vi "UHR-Fleezers Control (host) - 11.9.vi"() -> ()   [LabVIEW 2014] (continued)
                    tunnel: [w550 w565] -> w545
                    tunnel: w544 -> [_ w561]
                    frame False {
                      n310 = local read "Fish"() -> (w550:bool)
                      n311 = case shown="False" w550 {
                        tunnel: w551 -> [w552 _]
                        frame False {
                          n312 = property on="BD 1 Frequency 1 (MHz)" class="DigNum (strict)"("Val(Sgnl)"=w552) -> ()  [unwired: 2 in, 2 out]
                        }
                        frame True {
                        }
                      }
                    }
                    frame True {
                      w565 = FALSE ("Fish for Tether")
                      n313 = call <vilib>:"Beep.vi"() -> ()  [unwired: 3 in, 9 out]
                      n314 = Number To Decimal String(number=w561, width (-)=i16 1) -> (decimal integer string=w559:string)
                      n315 = Concatenate Strings("Formed tether in ", w559, " attempt(s)." ("string")) -> (w556:string)
                      n316 = local read "Messages"() -> (w563:string)
                      n317 = local write "Fish"(w565) -> ()
                      n318 = call "Update messages.vi"("Message to add"=w556, "Old message string"=w563) -> ("New message string"=w562:string)
                      n319 = local write "Messages"(w562) -> ()
                      n320 = Get Date/Time In Seconds() -> (seconds since 1Jan1904=→"Time tether formed":timestamp)
                      n321 = local read "Flow ON\nduring cal?"() -> (w553:bool)
                      n322 = property on="Sample Channel\nFlow" class="Bool (strict)"("Val(Sgnl)"=w553) -> (error out=w554:errorcluster)  [unwired: 2 in, 1 out]
                      n323 = case shown="\"2\", \"3\", \"4\", \"5\", \"6\"" "Then..." {
                        selector: "Then..." -> [_ w569 _ _]
                        tunnel: w566 -> [w568 _ _ _]
                        tunnel: w554 -> [_ _ _ _]
                        frame "1", Default {
                          n324 = property on="BD 1 Frequency 1 (MHz)" class="DigNum (strict)"("Val(Sgnl)"=w568) -> ()  [unwired: 2 in, 2 out]
                        }
                        frame "2", "3", "4", "5", "6" {
                          n325 = flat-sequence {
                            tunnel: w569 -> [w575]
                            frame #0 {
                              n326 = local read "Flow ON\nduring cal?"() -> (w570:bool)
                              n327 = property on="Sample Channel\nFlow" class="Bool (strict)"("Val(Sgnl)"=w570) -> ()  [unwired: 2 in, 2 out]
                              n328 = property on="Trap D (MHz)" class="DigNum (strict)"("Val(Sgnl)"="Move to D 1 (MHz)") -> ()  [unwired: 2 in, 2 out]
                            }
                            frame #1 {
                              n329 = local read "Wait Before Save (s)"() -> (w572:u32)
                              n330 = Multiply(x=u32 1000 ("milliseconds to wait"), y=w572) -> (x*y=w574:u32)
                              n331 = Wait (ms)(milliseconds to wait=w574) -> ()  [unwired: 1 out]
                            }
                            frame #2 {
                              n332 = case shown="\"5\", \"6\"" w575 {
                                selector: w575 -> [w578 w588 _]
                                frame "3", "4" {
                                n333 = flat-sequence {
                                tunnel: w578 -> [w579]
                                tunnel: [w579] -> w576
                                tunnel: [w581] -> w577
                                tunnel: w576 -> [w581]
                                tunnel: w577 -> [w585]
                                frame #0 {
                                n334 = property on="Green ON/Interlacing" class="Bool (strict)"("Val(Sgnl)"=TRUE ("Value (Signaling)")) -> ()  [unwired: 2 in, 2 out]
                                }
                                frame #1 {
                                n335 = Multiply(x="Wait Before Save (s)", y=u32 1000 ("x")) -> (x*y=w583:u32)
                                n336 = Wait (ms)(milliseconds to wait=w583) -> ()  [unwired: 1 out]
                                }
                                frame #2 {
                                n337 = property on="Start Saving" class="Bool (strict)"("Value"=TRUE ("Start Saving")) -> ()  [unwired: 2 in, 2 out]
                                n338 = case shown="\"4\"" w585 {
                                frame Default {
                                }
                                frame "4" {
                                n339 = property on="Fl. Triggered..." class="Bool (strict)"("Val(Sgnl)"=TRUE ("Value (Signaling)")) -> ()  [unwired: 2 in, 2 out]
                                }
                                }
                                }
                                }
                                }
                                frame "5", "6" {
                                n340 = stacked-sequence {
                                tunnel: w588 -> [_ _ _ _ _ _ w600]
                                frame #0 {
                                n341 = Replace Array Subset(array=u32[] [0] ("Index Values"), new element="Raster Set\nUpon Tether", index=0) -> (w589:u32[])
                                n342 = property on="Saved AOD Raster Scan Parameter Sets" class="Arr (strict)"("Index Values"=w589) -> ()  [unwired: 2 in, 2 out]
                                }
                                frame #1 {
                                n343 = Wait (ms)(milliseconds to wait=u32 500) -> ()  [unwired: 1 out]
                                }
                                frame #2 {
                                n344 = property on="Load parameters" class="Bool (strict)"("Val(Sgnl)"=TRUE ("Value (Signaling)")) -> ()  [unwired: 2 in, 2 out]
                                n345 = case shown="True" "Green ON during\nraster?" {
                                frame False {
                                }
                                frame True {
                                n346 = property on="Green ON/Interlacing" class="Bool (strict)"("Val(Sgnl)"=TRUE ("Value (Signaling)")) -> ()  [unwired: 2 in, 2 out]
                                }
                                }
                                }
                                frame #3 {
                                n347 = Wait (ms)(milliseconds to wait=u32 500) -> ()  [unwired: 1 out]
                                }
                                frame #4 {
                                n348 = property on="Trap Raster Scan" class="Bool (strict)"("Val(Sgnl)"=TRUE ("Value (Signaling)")) -> ()  [unwired: 2 in, 2 out]
                                }
                                frame #5 {
                                n349 = Wait (ms)(milliseconds to wait=u32 2000) -> ()  [unwired: 1 out]
                                }
                                frame #6 {
                                n350 = flat-sequence {
                                tunnel: w600 -> [w607]
                                frame #0 {
                                n351 = while {
                                stop <- w603 stop-if-true
                                n352 = local read "Raster Scanning..."() -> (w602:bool)
                                n353 = local read "Saving..."() -> (w605:bool)
                                n354 = Wait (ms)(milliseconds to wait=u32 100) -> ()  [unwired: 1 out]
                                n355 = Not(x=w605) -> (.not. x?=w604:bool)
                                n356 = Not(x=w602) -> (.not. x?=w601:bool)
                                n357 = And(x=w604, y=w601) -> (x .and. y?=w603:bool)
                                }
                                }
                                frame #1 {
                                n358 = local read "Tether"() -> (w608:bool)
                                n359 = case shown="True" w608 {
                                tunnel: w607 -> [_ w610]
                                frame False {
                                n360 = property on="Fish" class="Bool (strict)"("Val(Sgnl)"="Fish again after \nraster break?") -> ()  [unwired: 2 in, 2 out]
                                }
                                frame True {
                                n361 = stacked-sequence {
                                tunnel: w610 -> [_ w614 _ _ _ _ _ _]
                                frame #0 {
                                n362 = property on="Trap D (MHz)" class="DigNum (strict)"("Val(Sgnl)"="Move to D 2 (MHz)") -> ()  [unwired: 2 in, 2 out]
                                n363 = case shown="True" "Flow ON after\ntether testing?" {
                                frame False {
                                }
                                frame True {
                                n364 = property on="Sample Channel\nFlow" class="Bool (strict)"("Val(Sgnl)"=TRUE ("Value (Signaling)")) -> ()  [unwired: 2 in, 2 out]
                                }
                                }
                                }
                                frame #1 {
                                n365 = flat-sequence {
                                tunnel: w614 -> [w615]
                                frame #0 {
                                n366 = case shown="\"6\"" w615 {
                                frame Default {
                                }
                                frame "6" {
                                n367 = flat-sequence {
                                frame #0 {
                                n368 = Wait (ms)(milliseconds to wait=u32 500) -> ()  [unwired: 1 out]
                                }
                                frame #1 {
                                n369 = property on="Green ON/Interlacing" class="Bool (strict)"("Val(Sgnl)"=TRUE ("Green Laser ON/Interlacing")) -> ()  [unwired: 2 in, 2 out]
                                }
                                }
                                }
                                }
                                }
                                frame #1 {
                                n370 = case shown="True" "Save at end (5, 6)" {
                                selector: "Save at end (5, 6)" -> [_ w619]
                                frame False {
                                }
                                frame True {
                                n371 = flat-sequence {
                                tunnel: w619 -> [w621]
                                frame #0 {
                                n372 = Wait (ms)(milliseconds to wait=u32 500) -> ()  [unwired: 1 out]
                                }
                                frame #1 {
                                n373 = local write "Start Saving"(w621) -> ()
                                }
                                }
                                }
                                }
                                }
                                }
                                }
                                frame #2 {
                                n374 = local read "Bead Sep. Int. Time (s)"() -> (w624:dbl)
                                n375 = Multiply(x=w624, y=1000.0) -> (x*y=w623:dbl)
                                n376 = Wait (ms)(milliseconds to wait=w623) -> ()  [unwired: 1 out]
                                }
                                frame #3 {
                                n377 = property on="Remove Offset" class="Bool (strict)"("Val(Sgnl)"=TRUE ("Value (Signaling)")) -> ()  [unwired: 2 in, 2 out]
                                }
                                frame #4 {
                                n378 = property on="Read FX file" class="Bool (strict)"("Val(Sgnl)"=TRUE ("Value (Signaling)")) -> ()  [unwired: 2 in, 2 out]
                                }
                                frame #5 {
                                n379 = Wait (ms)(milliseconds to wait=u32 300) -> ()  [unwired: 1 out]
                                }
                                frame #6 {
                                n380 = local read "Bad fit error"() -> (w633:dbl)
                                n381 = local read "Fit offset"() -> (w636:dbl)
                                n382 = Greater Or Equal?(x=w633, y="Bad fit thresh") -> (x >= y?=→"Bad fit":bool)
                                n383 = Greater Or Equal?(x=w636, y="Fit offset thresh") -> (x >= y?=→"Multiple tether":bool)
                                n384 = local read "Hyst. error"() -> (w630:dbl)
                                n385 = Greater Or Equal?(x=w630, y="Hysteresis thresh") -> (x >= y?=→"Hysteresis":bool)
                                }
                                frame #7 {
                                w641 = 0
                                n386 = local read "Bad fit error"() -> (w643:dbl)
                                n387 = local read "Hyst. error"() -> (w642:dbl)
                                n388 = local read "Fit offset"() -> (w644:dbl)
                                n389 = local read "Multiple tether"() -> (w650:bool)
                                n390 = local read "Hysteresis"() -> (w648:bool)
                                n391 = local read "Bad fit"() -> (w649:bool)
                                n392 = Not(x=w648) -> (.not. x?=w640:bool)
                                n393 = Not(x=w649) -> (.not. x?=w646:bool)
                                n394 = Greater?(x=w644, y=w641) -> (0:w639:bool)
                                n395 = Greater?(x=w643, y=w641) -> (0:w638:bool)
                                n396 = Greater?(x=w642, y=w641) -> (0:w637:bool)
                                n397 = Not(x=w650) -> (.not. x?=w647:bool)
                                n398 = Compound Arithmetic op=AND(w647, w646, w640, w639, w638, w637) -> (w645:bool)
                                "Good tether" <- w645
                                n399 = case shown="True" w645 {
                                frame False {
                                }
                                frame True {
                                n400 = call <vilib>:"Beep.vi"("use system alert? (T)"=FALSE, "duration (msec)"=u32 200, "frequency (Hz)"=u32 2000) -> ()  [unwired: 9 in]
                                }
                                }
                                }
                                }
                                }
                                }
                                }
                                }
                                }
                                }
                                }
                                frame "2", Default {
                                }
                              }
                            }
                            frame #3 {
                              n401 = local read "Multiple tether"() -> (w656:bool)
                              n402 = And(x="Break multiple", y=w656) -> (x .and. y?=w654:bool)
                              n403 = case shown="True" w654 {
                                frame False {
                                }
                                frame True {
                                n404 = stacked-sequence {
                                frame #0 {
                                n405 = property on="Trap D (MHz)" class="DigNum (strict)"("Val(Sgnl)"="Trap D to \nbreak (MHz)") -> ()  [unwired: 2 in, 2 out]
                                }
                                frame #1 {
                                n406 = case shown="True" "Fish after\nmultiple break" {
                                frame False {
                                }
                                frame True {
                                n407 = while {
                                stop <- w661 stop-if-true
                                n408 = local read "Multiple tether"() -> (w663:bool)
                                n409 = local read "Fish"() -> (w660:bool)
                                n410 = local read "Stop All"() -> (w659:bool)
                                n411 = Wait (ms)(milliseconds to wait=u32 100) -> ()  [unwired: 1 out]
                                n412 = Not(x=w663) -> (.not. x?=w662:bool)
                                n413 = Compound Arithmetic op=OR(w659, w662, w660) -> (w661:bool)
                                }
                                }
                                }
                                }
                                frame #2 {
                                n414 = local read "Fish after\nmultiple break"() -> (w668:bool)
                                n415 = local read "Stage Moving"() -> (w667:bool)
                                n416 = Not(x=w667) -> (.not. x?=w665:bool)
                                n417 = And(x=w668, y=w665) -> (x .and. y?=w666:bool)
                                n418 = property on="Fish" class="Bool (strict)"("Val(Sgnl)"=w666) -> ()  [unwired: 2 in, 2 out]
                                }
                                }
                                }
                              }
                            }
                            frame #4 {
                              n419 = local read "Bad fit"() -> (w670:bool)
                              n420 = And(x="Break bad fit", y=w670) -> (x .and. y?=w669:bool)
                              n421 = case shown="True" w669 {
                                frame False {
                                }
                                frame True {
                                n422 = stacked-sequence {
                                frame #0 {
                                n423 = local read "Trap D to \nbreak (MHz)"() -> (w672:dbl)
                                n424 = property on="Trap D (MHz)" class="DigNum (strict)"("Val(Sgnl)"=w672) -> ()  [unwired: 2 in, 2 out]
                                }
                                frame #1 {
                                n425 = case shown="True" "Fish after\nbad fit break?" {
                                frame False {
                                }
                                frame True {
                                n426 = while {
                                stop <- w676 stop-if-true
                                n427 = local read "Stop All"() -> (w674:bool)
                                n428 = local read "Bad fit"() -> (w675:bool)
                                n429 = local read "Fish"() -> (w677:bool)
                                n430 = Not(x=w675) -> (.not. x?=w678:bool)
                                n431 = Wait (ms)(milliseconds to wait=u32 100) -> ()  [unwired: 1 out]
                                n432 = Compound Arithmetic op=OR(w674, w678, w677) -> (w676:bool)
                                }
                                }
                                }
                                }
                                frame #2 {
                                n433 = local read "Fish after\nbad fit break?"() -> (w680:bool)
                                n434 = local read "Stage Moving"() -> (w683:bool)
                                n435 = Not(x=w683) -> (.not. x?=w682:bool)
                                n436 = And(x=w680, y=w682) -> (x .and. y?=w681:bool)
                                n437 = property on="Fish" class="Bool (strict)"("Val(Sgnl)"=w681) -> ()  [unwired: 2 in, 2 out]
                                }
                                }
                                }
                              }
                            }
                            frame #5 {
                              n438 = local read "Hysteresis"() -> (w685:bool)
                              n439 = And(x="Break hyst", y=w685) -> (x .and. y?=w684:bool)
                              n440 = case shown="True" w684 {
                                frame False {
                                }
                                frame True {
                                n441 = stacked-sequence {
                                frame #0 {
                                n442 = local read "Trap D to \nbreak (MHz)"() -> (w687:dbl)
                                n443 = property on="Trap D (MHz)" class="DigNum (strict)"("Val(Sgnl)"=w687) -> ()  [unwired: 2 in, 2 out]
                                }
                                frame #1 {
                                n444 = case shown="True" "Fish ater hyst?" {
                                frame False {
                                }
                                frame True {
                                n445 = while {
                                stop <- w693 stop-if-true
                                n446 = local read "Hysteresis"() -> (w692:bool)
                                n447 = local read "Stop All"() -> (w689:bool)
                                n448 = local read "Fish"() -> (w690:bool)
                                n449 = Wait (ms)(milliseconds to wait=u32 100) -> ()  [unwired: 1 out]
                                n450 = Not(x=w692) -> (.not. x?=w691:bool)
                                n451 = Compound Arithmetic op=OR(w689, w691, w690) -> (w693:bool)
                                }
                                }
                                }
                                }
                                frame #2 {
                                n452 = local read "Fish ater hyst?"() -> (w698:bool)
                                n453 = local read "Stage Moving"() -> (w697:bool)
                                n454 = Not(x=w697) -> (.not. x?=w696:bool)
                                n455 = And(x=w698, y=w696) -> (x .and. y?=w695:bool)
                                n456 = property on="Fish" class="Bool (strict)"("Val(Sgnl)"=w695) -> ()  [unwired: 2 in, 2 out]
                                }
                                }
                                }
                              }
                            }
                            frame #6 {
                              n457 = local read "Good tether"() -> (w699:bool)
                              n458 = case shown="True" w699 {
                                frame False {
                                }
                                frame True {
                                n459 = case shown="\"1\"" "If good, then:" {
                                frame "0", Default {
                                }
                                frame "1" {
                                n460 = property on="Force FB Script" class="Bool (strict)"("Val(Sgnl)"=TRUE ("Value (Signaling)")) -> ()  [unwired: 2 in, 2 out]
                                }
                                }
                                }
                              }
                            }
                          }
                        }
                        frame "7" {
                          n461 = property on="Force FB Script" class="Bool (strict)"("Val(Sgnl)"=TRUE ("Value (Signaling)")) -> ()  [unwired: 2 in, 2 out]
                        }
                        frame "8" {
                          n462 = property on="Fixed Traps Script" class="Bool (strict)"("Val(Sgnl)"=TRUE ("Value (Signaling)")) -> ()  [unwired: 2 in, 2 out]
                        }
                      }
                      "Tether" <- "Tether Alarm?"
                    }
                  }
                }
                frame #2 {
                  n463 = local read "Oscillate Set 1"() -> (w709:bool)
                  n464 = local read "Stop All"() -> (w707:bool)
                  n465 = Or(x=w709, y=w704) -> (x .or. y?=w706:bool)
                  n466 = Not(x=w706) -> (.not. x?=w708:bool)
                  n467 = Compound Arithmetic op=OR(w707, w708) -> (w705:bool)
                }
              }
              n468 = node-c288() -> ()  [unwired: 2 out]
            }
            n469 = node-c288(w459) -> ()  [unwired: 1 out]
          }
        }
      }
      event "Fl. Triggered...": Value Change {
        n470 = event-data() -> ()  [unwired: 7 out]
        n471 = case shown="True" "Fl. Triggered..." {
          frame False {
          }
          frame True {
            n472 = node-c288() -> (w720:T21)  [unwired: 4 out]
            n473 = timed-loop {
              timing: w720 -> [_]
              timing-out: [_] -> w719
              tunnel: "Action" -> [w728]
              shift-right: [w725] -> _
              shift-left: u8 255 -> [w727]
              shift-right: [w722] -> _
              shift-left: 255 -> [w724]
              stop <- w721 stop-if-true
              # "Reset confocal spot"
              n474 = node-c288() -> ()  [unwired: 2 out]
              n475 = flat-sequence {
                tunnel: w728 -> [w748]
                tunnel: w727 -> [w747]
                tunnel: [w746] -> w726
                tunnel: w724 -> [w733]
                tunnel: [w732] -> w723
                tunnel: [w1132] -> w721
                tunnel: w726 -> [w1131]
                tunnel: [w1131] -> w725
                tunnel: [w1130] -> w722
                tunnel: w723 -> [w1130]
                frame #0 {
                  n476 = local read "Delta Fl. 2"() -> (w745:dbl)
                  n477 = local read "Delta Fl. 1"() -> (w740:dbl)
                  n478 = Multiply(x="Fl. D Thresh. (kHz)", y=1000.0) -> (x*y=w735:dbl)
                  n479 = Select(t=w740, s="APD to Watch", f=w745) -> (s? t:f=w736:dbl)
                  n480 = Greater?(x=w736, y=w735) -> (0:w741:bool)
                  n481 = Or(x="Force Yank", y=w741) -> (x .or. y?=w739:bool)
                  n482 = And(x=w739, y="Yank when?") -> (x .and. y?=w737:bool)
                  n483 = case shown="False" w737 {
                    tunnel: w748 -> [w751 w954]
                    tunnel: w747 -> [w753 w950]
                    tunnel: [w753 w948] -> w746
                    tunnel: w736 -> [w759 _]
                    tunnel: w735 -> [w758 _]
                    tunnel: "Force Yank" -> [w756 _]
                    tunnel: w733 -> [w755 w947]
                    tunnel: [w754 w947] -> w732
                    frame False {
                      n484 = Negate(x=w758) -> (-x=w750:dbl)
                      n485 = local write "Fl. High"(TRUE ("Fl. High")) -> ()
                      n486 = Less?(x=w759, y=w750) -> (x < y?=w757:bool)
                      n487 = Or(x=w756, y=w757) -> (x .or. y?=w752:bool)
                      n488 = case shown="True" w752 {
                        tunnel: w755 -> [w760 w770]
                        tunnel: [w760 w769] -> w754
                        tunnel: w751 -> [_ w768]
                        frame False {
                        }
                        frame True {
                          n489 = flat-sequence {
                            tunnel: w770 -> [w776]
                            tunnel: w768 -> [w773]
                            tunnel: [w775] -> w767
                            tunnel: [w774] -> w766
                            tunnel: [w773] -> w765
                            tunnel: w764 -> [w772]
                            tunnel: [w772] -> w763
                            tunnel: w762 -> [w771]
                            tunnel: [w771] -> w761
                            tunnel: [w848] -> w769
                            tunnel: w767 -> [w848]
                            tunnel: w766 -> [w847]
                            tunnel: w765 -> [w846]
                            tunnel: w763 -> [w845]
                            tunnel: w761 -> [w844]
                            frame #0 {
                              n490 = call <vilib>:"Beep.vi"() -> ()  [unwired: 12 in]
                              n491 = local write "Waiting"(FALSE ("Waiting")) -> ()
                              n492 = Increment(x=w776) -> (x+1=w775:i32)
                              n493 = case shown="\"Yank\"" w773 {
                                tunnel: w775 -> [_ w781 _]
                                frame "Alarm", Default {
                                }
                                frame "Yank" {
                                n494 = flat-sequence {
                                tunnel: w781 -> [w784]
                                tunnel: [w783] -> w780
                                tunnel: [w782] -> w779
                                tunnel: w780 -> [w794]
                                tunnel: w779 -> [w795]
                                frame #0 {
                                n495 = local read "Yank Delay (s)"() -> (w787:dbl)
                                n496 = local read "N Array El"() -> (w782:u8)
                                n497 = Quotient & Remainder(x=w784, y=w782) -> (x-y*floor(x/y)=w783:i32)  [unwired: 1 out]
                                n498 = Multiply(x=w787, y=1000.0) -> (x*y=w785:dbl)
                                n499 = Wait (ms)(milliseconds to wait=w785) -> ()  [unwired: 1 out]
                                }
                                frame #1 {
                                n500 = local read "Yank to which?"() -> (w789:bool)
                                n501 = local read "Random Choice"() -> (w799:bool)
                                n502 = local read "Yank to Trap D (MHz)"() -> (w792:dbl[])
                                n503 = local read "Yank to SP"() -> (w793:dbl[])
                                n504 = Random Number (0-1)() -> (number: 0 to 1=w798:dbl)
                                n505 = Multiply(x=w795, y=w798) -> (x*y=w797:dbl)
                                n506 = Round Toward -Infinity(1:w797) -> (0:w796:dbl)
                                n507 = Select(t=w796, s=w799, f=w794) -> (s? t:f=w790:dbl)
                                n508 = Select(t=w792, s=w789, f=w793) -> (s? t:f=w791:dbl[])
                                n509 = Index Array(array=w791, index=w790) -> (element=w788:dbl)
                                n510 = case shown="False" w789 {
                                tunnel: w788 -> [w800 w828]
                                frame False {
                                n511 = flat-sequence {
                                tunnel: w800 -> [w801]
                                frame #0 {
                                n512 = property on="Trap Pos FB SP" class="DigNum (strict)"("Val(Sgnl)"=w801) -> ()  [unwired: 2 in, 2 out]
                                }
                                frame #1 {
                                n513 = Wait (ms)(milliseconds to wait=u32 700) -> ()  [unwired: 1 out]
                                }
                                frame #2 {
                                n514 = local read "Action (%)"() -> (w806:dbl)
                                n515 = Absolute Value(x=w806) -> (abs(x)=w805:dbl)
                                n516 = Greater?(x=w805, y=70.0) -> (0:w803:bool)
                                n517 = property on="Remove Action Offset" class="Bool (strict)"("Val(Sgnl)"=w803) -> ()  [unwired: 2 in, 2 out]
                                }
                                frame #3 {
                                n518 = for {
                                N: 4 -> [_]
                                n519 = flat-sequence {
                                frame #0 {
                                n520 = Wait (ms)(milliseconds to wait=u32 500) -> ()  [unwired: 1 out]
                                }
                                frame #1 {
                                n521 = local read "Action (%)"() -> (w812:dbl)
                                n522 = Absolute Value(x=w812) -> (abs(x)=w811:dbl)
                                n523 = Greater?(x=w811, y=70.0) -> (0:w809:bool)
                                n524 = property on="Remove Action Offset" class="Bool (strict)"("Val(Sgnl)"=w809) -> ()  [unwired: 2 in, 2 out]
                                }
                                }
                                }
                                }
                                frame #4 {
                                n525 = Wait (ms)(milliseconds to wait=u32 500) -> ()  [unwired: 1 out]
                                }
                                frame #5 {
                                n526 = local read "Mean"() -> (w820:dbl)
                                n527 = Greater?(x=w820, y=11.0) -> (0:w814:bool)
                                n528 = Not(x=w814) -> (.not. x?=w815:bool)
                                n529 = And(x=w815, y="Shift confocal") -> (x .and. y?=w817:bool)
                                n530 = And(x=w814, y="Shift confocal") -> (x .and. y?=w818:bool)
                                n531 = case shown="True" w818 {
                                frame False {
                                }
                                frame True {
                                n532 = local read "Confocal Y 2 (V)"() -> (w824:dbl)
                                n533 = local read "Confocal X 2 (V)"() -> (w823:dbl)
                                n534 = property on="AO1" class="Slide (strict)"("Val(Sgnl)"=w824) -> ()  [unwired: 2 in, 2 out]
                                n535 = property on="AO2" class="Slide (strict)"("Val(Sgnl)"=w823) -> ()  [unwired: 2 in, 2 out]
                                }
                                }
                                n536 = case shown="True" w817 {
                                frame False {
                                }
                                frame True {
                                n537 = local read "Confocal Y 1 (V)"() -> (w822:dbl)
                                n538 = local read "Confocal X 1 (V)"() -> (w821:dbl)
                                n539 = property on="AO1" class="Slide (strict)"("Val(Sgnl)"=w822) -> ()  [unwired: 2 in, 2 out]
                                n540 = property on="AO2" class="Slide (strict)"("Val(Sgnl)"=w821) -> ()  [unwired: 2 in, 2 out]
                                }
                                }
                                }
                                frame #6 {
                                n541 = Wait (ms)(milliseconds to wait=u32 1500) -> ()  [unwired: 1 out]
                                }
                                frame #7 {
                                n542 = property on="Rem fb disp offset" class="Bool (strict)"("Val(Sgnl)"=TRUE ("Value (Signaling)")) -> ()  [unwired: 2 in, 2 out]
                                n543 = property on="Remove Offset" class="Bool (strict)"("Val(Sgnl)"=TRUE ("Value (Signaling)")) -> ()  [unwired: 2 in, 2 out]
                                }
                                }
                                }
                                frame True {
                                n544 = flat-sequence {
                                tunnel: w828 -> [w829]
                                frame #0 {
                                n545 = property on="Trap D (MHz)" class="DigNum (strict)"("Val(Sgnl)"=w829) -> ()  [unwired: 2 in, 2 out]
                                }
                                frame #1 {
                                n546 = Wait (ms)(milliseconds to wait=u32 500) -> ()  [unwired: 1 out]
                                }
                                frame #2 {
                                n547 = local read "Shift confocal"() -> (w835:bool)
                                n548 = local read "Mean"() -> (w837:dbl)
                                n549 = Greater?(x=w837, y=11.0) -> (0:w834:bool)
                                n550 = Not(x=w834) -> (.not. x?=w833:bool)
                                n551 = And(x=w833, y=w835) -> (x .and. y?=w831:bool)
                                n552 = And(x=w834, y=w835) -> (x .and. y?=w832:bool)
                                n553 = case shown="True" w832 {
                                frame False {
                                }
                                frame True {
                                n554 = local read "Confocal Y 2 (V)"() -> (w841:dbl)
                                n555 = local read "Confocal X 2 (V)"() -> (w840:dbl)
                                n556 = property on="AO2" class="Slide (strict)"("Val(Sgnl)"=w840) -> ()  [unwired: 2 in, 2 out]
                                n557 = property on="AO1" class="Slide (strict)"("Val(Sgnl)"=w841) -> ()  [unwired: 2 in, 2 out]
                                }
                                }
                                n558 = case shown="True" w831 {
                                frame False {
                                }
                                frame True {
                                n559 = local read "Confocal X 1 (V)"() -> (w838:dbl)
                                n560 = local read "Confocal Y 1 (V)"() -> (w839:dbl)
                                n561 = property on="AO2" class="Slide (strict)"("Val(Sgnl)"=w838) -> ()  [unwired: 2 in, 2 out]
                                n562 = property on="AO1" class="Slide (strict)"("Val(Sgnl)"=w839) -> ()  [unwired: 2 in, 2 out]
                                }
                                }
                                }
                                }
                                }
                                }
                                }
                                }
                                }
                                frame "Image" {
                                n563 = property on="Confocal\nImage" class="Bool (strict)"("Val(Sgnl)"=TRUE ("Value (Signaling)")) -> ()  [unwired: 2 in, 2 out]
                                }
                              }
                              n564 = local write "Fl. High"(FALSE ("Fl. High")) -> ()
                              n565 = local read "Time (s)"() -> (w774:dbl)
                            }
                            frame #1 {
                              n566 = case shown="True" "Auto F Reset" {
                                tunnel: w847 -> [_ w852]
                                tunnel: w846 -> [_ w851]
                                tunnel: w845 -> [_ w850]
                                tunnel: w844 -> [_ w849]
                                frame False {
                                }
                                frame True {
                                n567 = node-c288() -> (w854:T21)  [unwired: 4 in]
                                n568 = timed-loop {
                                timing: w854 -> [_]
                                timing-out: [_] -> w853
                                tunnel: w852 -> [w859]
                                tunnel: w851 -> [w858]
                                tunnel: w850 -> [w857]
                                tunnel: w849 -> [w856]
                                stop <- w855 stop-if-true
                                n569 = node-c288() -> ()  [unwired: 1 in, 1 out]
                                n570 = local read "APD to Watch"() -> (w869:bool)
                                n571 = local read "Fl. D Thresh. (kHz)"() -> (w868:dbl)
                                n572 = local read "Delta Fl. 1"() -> (w870:dbl)
                                n573 = local read "Delta Fl. 2"() -> (w871:dbl)
                                n574 = local read "Fl. Triggered..."() -> (w862:bool)
                                n575 = local read "Stop All"() -> (w863:bool)
                                n576 = local read "Reset Force"() -> (w861:bool)
                                n577 = Multiply(x=w868, y=1000.0) -> (x*y=w866:dbl)
                                n578 = Not(x=w862) -> (.not. x?=w860:bool)
                                n579 = Select(t=w870, s=w869, f=w871) -> (s? t:f=w865:dbl)
                                n580 = Greater?(x=w865, y=w866) -> (0:w864:bool)
                                n581 = Compound Arithmetic op=OR(w864, w863, w860, w861) -> (w855:bool)
                                n582 = case shown="True" w855 {
                                tunnel: w859 -> [_ w875]
                                tunnel: w858 -> [_ w879]
                                tunnel: w857 -> [_ w878]
                                tunnel: w856 -> [_ w877]
                                frame False {
                                }
                                frame True {
                                n583 = case shown="\"Yank\"" w879 {
                                tunnel: w878 -> [_ w889]
                                tunnel: w877 -> [_ w887]
                                frame "Image", Default {
                                }
                                frame "Yank" {
                                n584 = flat-sequence {
                                tunnel: [w892] -> w890
                                tunnel: w889 -> [w892]
                                tunnel: [w891] -> w888
                                tunnel: w887 -> [w891]
                                tunnel: w890 -> [w898]
                                tunnel: w888 -> [w896]
                                frame #0 {
                                n585 = local read "Yank Delay (s)"() -> (w895:dbl)
                                n586 = Multiply(x=w895, y=1000.0) -> (x*y=w893:dbl)
                                n587 = Wait (ms)(milliseconds to wait=w893) -> ()  [unwired: 1 out]
                                }
                                frame #1 {
                                n588 = local read "Yank to which?"() -> (w897:bool)
                                n589 = case shown="False" w897 {
                                tunnel: w898 -> [_ w927]
                                tunnel: w896 -> [w899 _]
                                frame False {
                                n590 = flat-sequence {
                                tunnel: w899 -> [w900]
                                frame #0 {
                                n591 = property on="Trap Pos FB SP" class="DigNum (strict)"("Val(Sgnl)"=w900) -> ()  [unwired: 2 in, 2 out]
                                }
                                frame #1 {
                                n592 = Wait (ms)(milliseconds to wait=u32 700) -> ()  [unwired: 1 out]
                                }
                                frame #2 {
                                n593 = local read "Action (%)"() -> (w905:dbl)
                                n594 = Absolute Value(x=w905) -> (abs(x)=w904:dbl)
                                n595 = Greater?(x=w904, y=70.0) -> (0:w902:bool)
                                n596 = property on="Remove Action Offset" class="Bool (strict)"("Val(Sgnl)"=w902) -> ()  [unwired: 2 in, 2 out]
                                }
                                frame #3 {
                                n597 = for {
                                N: 4 -> [_]
                                n598 = flat-sequence {
                                frame #0 {
                                n599 = Wait (ms)(milliseconds to wait=u32 500) -> ()  [unwired: 1 out]
                                }
                                frame #1 {
                                n600 = local read "Action (%)"() -> (w911:dbl)
                                n601 = Absolute Value(x=w911) -> (abs(x)=w910:dbl)
                                n602 = Greater?(x=w910, y=70.0) -> (0:w908:bool)
                                n603 = property on="Remove Action Offset" class="Bool (strict)"("Val(Sgnl)"=w908) -> ()  [unwired: 2 in, 2 out]
                                }
                                }
                                }
                                }
                                frame #4 {
                                n604 = Wait (ms)(milliseconds to wait=u32 500) -> ()  [unwired: 1 out]
                                }
                                frame #5 {
                                n605 = local read "Shift confocal"() -> (w916:bool)
                                n606 = local read "Mean"() -> (w919:dbl)
                                n607 = Greater?(x=w919, y=11.0) -> (0:w915:bool)
                                n608 = Not(x=w915) -> (.not. x?=w914:bool)
                                n609 = And(x=w915, y=w916) -> (x .and. y?=w917:bool)
                                n610 = And(x=w914, y=w916) -> (x .and. y?=w913:bool)
                                n611 = case shown="True" w917 {
                                frame False {
                                }
                                frame True {
                                n612 = local read "Confocal X 2 (V)"() -> (w922:dbl)
                                n613 = local read "Confocal Y 2 (V)"() -> (w923:dbl)
                                n614 = property on="AO2" class="Slide (strict)"("Val(Sgnl)"=w922) -> ()  [unwired: 2 in, 2 out]
                                n615 = property on="AO1" class="Slide (strict)"("Val(Sgnl)"=w923) -> ()  [unwired: 2 in, 2 out]
                                }
                                }
                                n616 = case shown="True" w913 {
                                frame False {
                                }
                                frame True {
                                n617 = local read "Confocal Y 1 (V)"() -> (w921:dbl)
                                n618 = local read "Confocal X 1 (V)"() -> (w920:dbl)
                                n619 = property on="AO1" class="Slide (strict)"("Val(Sgnl)"=w921) -> ()  [unwired: 2 in, 2 out]
                                n620 = property on="AO2" class="Slide (strict)"("Val(Sgnl)"=w920) -> ()  [unwired: 2 in, 2 out]
                                }
                                }
                                }
                                frame #6 {
                                n621 = Wait (ms)(milliseconds to wait=u32 1500) -> ()  [unwired: 1 out]
                                }
                                frame #7 {
                                n622 = property on="Remove Offset" class="Bool (strict)"("Val(Sgnl)"=TRUE ("Value (Signaling)")) -> ()  [unwired: 2 in, 2 out]
                                n623 = property on="Rem fb disp offset" class="Bool (strict)"("Val(Sgnl)"=TRUE ("Value (Signaling)")) -> ()  [unwired: 2 in, 2 out]
                                }
                                }
                                }
                                frame True {
                                n624 = flat-sequence {
                                tunnel: w927 -> [w928]
                                frame #0 {
                                n625 = property on="Trap D (MHz)" class="DigNum (strict)"("Val(Sgnl)"=w928) -> ()  [unwired: 2 in, 2 out]
                                }
                                frame #1 {
                                n626 = Wait (ms)(milliseconds to wait=u32 500) -> ()  [unwired: 1 out]
                                }
                                frame #2 {
                                n627 = local read "Shift confocal"() -> (w934:bool)
                                n628 = local read "Mean"() -> (w935:dbl)
                                n629 = Greater?(x=w935, y=11.0) -> (0:w933:bool)
                                n630 = And(x=w933, y=w934) -> (x .and. y?=w931:bool)
                                n631 = Not(x=w933) -> (.not. x?=w932:bool)
                                n632 = And(x=w932, y=w934) -> (x .and. y?=w930:bool)
                                n633 = case shown="True" w931 {
                                frame False {
                                }
                                frame True {
                                n634 = local read "Confocal Y 2 (V)"() -> (w940:dbl)
                                n635 = local read "Confocal X 2 (V)"() -> (w939:dbl)
                                n636 = property on="AO1" class="Slide (strict)"("Val(Sgnl)"=w940) -> ()  [unwired: 2 in, 2 out]
                                n637 = property on="AO2" class="Slide (strict)"("Val(Sgnl)"=w939) -> ()  [unwired: 2 in, 2 out]
                                }
                                }
                                n638 = case shown="True" w930 {
                                frame False {
                                }
                                frame True {
                                n639 = local read "Confocal Y 1 (V)"() -> (w938:dbl)
                                n640 = local read "Confocal X 1 (V)"() -> (w937:dbl)
                                n641 = property on="AO2" class="Slide (strict)"("Val(Sgnl)"=w937) -> ()  [unwired: 2 in, 2 out]
                                n642 = property on="AO1" class="Slide (strict)"("Val(Sgnl)"=w938) -> ()  [unwired: 2 in, 2 out]
                                }
                                }
                                }
                                }
                                }
                                }
                                }
                                }
                                }
                                }
                                n643 = local read "Time (s)"() -> (w874:dbl)
                                n644 = Subtract(x=w875, y=w874) -> (x-y=w886:dbl)
                                n645 = Number To Decimal String(number=w886, width (-)=i16 0) -> (decimal integer string=w884:string)
                                n646 = Concatenate Strings(w884, " s fluorescence event") -> (w881:string)
                                n647 = local read "Messages"() -> (w882:string)
                                n648 = local write "Duration (s)"(w886) -> ()
                                n649 = call "Update messages.vi"("Message to add"=w881, "Old message string"=w882) -> ("New message string"=w880:string)
                                n650 = local write "Messages"(w880) -> ()
                                n651 = call <vilib>:"Beep.vi"() -> ()  [unwired: 12 in]
                                n652 = local write "Reset Force"(FALSE ("Force Reset")) -> ()
                                n653 = local write "Fl. High"(TRUE ("Fl. High")) -> ()
                                n654 = local write "Waiting"(TRUE ("Waiting")) -> ()
                                }
                                }
                                n655 = node-c288() -> ()  [unwired: 1 in, 1 out]
                                }
                                n656 = node-c288(w853) -> ()  [unwired: 1 out]
                                }
                              }
                            }
                          }
                          n657 = local read "Trap Pos FB SP"() -> (w762:fxp<+/-,16,1>)
                          n658 = local read "Trap D (MHz)"() -> (w764:dbl)
                        }
                      }
                    }
                    frame True {
                      n659 = flat-sequence {
                        tunnel: w951 -> [w961]
                        tunnel: [w961] -> w955
                        tunnel: w954 -> [w960]
                        tunnel: [w960] -> w953
                        tunnel: [w959] -> w952
                        tunnel: w950 -> [w958]
                        tunnel: [w957] -> w949
                        tunnel: w946 -> [w956]
                        tunnel: [w956] -> w945
                        tunnel: w955 -> [w1033]
                        tunnel: w953 -> [w1032]
                        tunnel: w952 -> [w1031]
                        tunnel: w949 -> [w1030]
                        tunnel: w945 -> [w1029]
                        tunnel: [w1030] -> w948
                        frame #0 {
                          n660 = call <vilib>:"Beep.vi"() -> ()  [unwired: 3 in, 9 out]
                          n661 = local write "Waiting"(FALSE ("Waiting")) -> ()
                          n662 = Increment(x=w958) -> (x+1=w957:u8)
                          n663 = case shown="\"Image\"" w960 {
                            tunnel: w957 -> [_ _ w967 _]
                            frame "Image" {
                              n664 = property on="Confocal\nImage" class="Bool (strict)"("Val(Sgnl)"=TRUE ("Value (Signaling)")) -> ()  [unwired: 2 in, 2 out]
                            }
                            frame "Alarm", Default {
                            }
                            frame "Yank" {
                              n665 = flat-sequence {
                                tunnel: w967 -> [w970]
                                tunnel: [w969] -> w966
                                tunnel: ["N Array El"] -> w965
                                tunnel: w966 -> [w984]
                                tunnel: w965 -> [w980]
                                frame #0 {
                                n666 = Multiply(x="Yank Delay (s)", y=1000.0) -> (x*y=w973:dbl)
                                n667 = Quotient & Remainder(x=w970, y="N Array El") -> (x-y*floor(x/y)=w969:u8)  [unwired: 1 out]
                                n668 = Wait (ms)(milliseconds to wait=w973) -> ()  [unwired: 1 out]
                                }
                                frame #1 {
                                n669 = Random Number (0-1)() -> (number: 0 to 1=w981:dbl)
                                n670 = Multiply(x=w980, y=w981) -> (x*y=w979:dbl)
                                n671 = Round Toward -Infinity(1:w979) -> (0:w978:dbl)
